vi "Setup UI.vi"(8 "error in (no error)":errorcluster, 10 "Set UI to input? (F)":bool, 11 "Lockin SR830 in":refnum<class "Lockin SR830.lvclass">) -> (0 "error out":errorcluster, 3 "Lockin SR830 out":refnum<class "Lockin SR830.lvclass">)   [LabVIEW 2009, in "Lockin SR830.lvclass"]
doc: "Setup UI constructs an object -- populates its member data -- from a front panel the user can see. The VI should be as simple as possible so that a UI loop can poll it continuously for updates. \n\nThe VI is designed to be used as a subPanel within another VI. Wire true to \"Set UI to input\" only on the first call, just after inserting this VI into a subPanel, to populate its controls with the class's current values.\n\nSetup UI is distinct from the class constructor. Class constructors are not polymorphic, yet configure dialogs need to configure objects without knowing their type -- and polymorphism is the necessary solution. Thus, Setup UI is a polymorphic class constructor. This continously polled \"Setup UI\" concept is a kludge: a better idea would be an XControl, but those require a steeper learning curve."
uses:
  Lockin SR830.lvclass
  Utility Classes/Readable/Readable.lvclass
panel:
  in  "Lockin Model":bool=TRUE
  # "Lockin Setup"
  # "SR810"
  # "SR830"
  # "GPIB #8"
  # "GPIB #9"
  # "Take data from\n(X,Y) channels"
  # "Take data from\ndisplay screens 1 & 2"
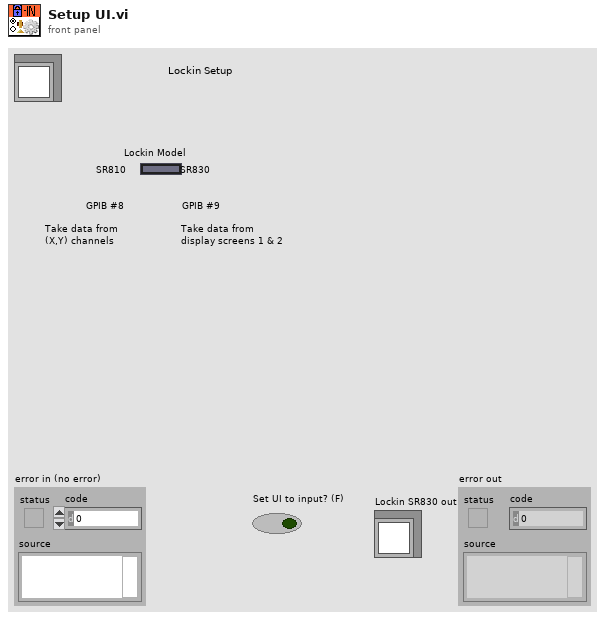
[diagram p1: front panel]
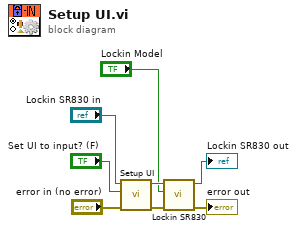
[diagram p0: block diagram]
diagram:
  n1 = call-parent "Setup UI.vi"("error in (no error)"="error in (no error)", "Set UI to input? (F)"="Set UI to input? (F)", "Instrument in"="Lockin SR830 in") -> ("error out"=w2:errorcluster, "Instrument out"=w5:refnum<class "Lockin SR830.lvclass">)  [unwired: 7 out]
  n2 = call "Lockin SR830.vi"("error in (no error)"=w2, "Is SR830? (T)"="Lockin Model", "Lockin SR830 in"=w5) -> ("error out"=→"error out":errorcluster, "Lockin SR830 out"=→"Lockin SR830 out":refnum<class "Lockin SR830.lvclass">)  [unwired: 7 out]
